vi "Manipulator Panel - UNTOUCHED.vi"() -> ()   [LabVIEW 2012]
uses:
  <vilib>/Platform/TimedLoop/XDataNode/timing_clust.ctl
  <vilib>/Platform/TimedLoop/XDataNode/nitl_modes.ctl
  <vilib>/Platform/TimedLoop/XDataNode/wakeup.ctl
  <vilib>/Platform/TimedLoop/XDataNode/XDataNode.xnode
  <vilib>/Platform/TimedLoop/XDataNode/XDNodeRunTimeDep.lvlib
panel:
  out "Active":bool
  out "Reset":bool
  in  "TCPConRef":refnum<k5>
  out "Turning off in":dbl=10.0
  in  "Power switch\nmanipulator":bool
  in  "Arm Rotate ccw":bool
  in  "Arm Rotate cw":bool
  in  "Claw close":bool
  in  "Claw open":bool
  in  "Arm right":bool
  in  "Arm left":bool
  in  "Lower arm down":bool
  in  "Lower arm up":bool
  in  "Upper arm down":bool
  in  "Upper arm up":bool
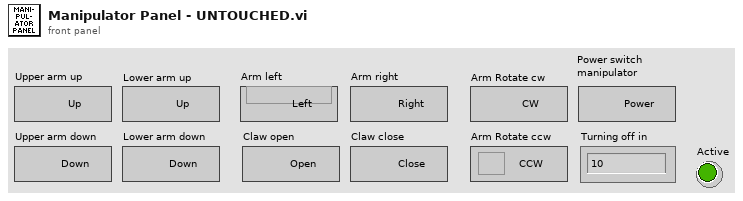
[diagram p1: front panel]
types:
  T1 = typedef "XDNodeRunTimeDep.lvlib/timing_clust.ctl" = cluster{"Expected End [f-1]":u64, "Actual End [f-1]":u64, "Finished Late? [f-1]":bool, "Expected End [i-1]":u64, "Actual End [i-1]":u64, "Finished Late? [i-1]":bool, "Expected Start [i]":u64, "Actual Start [i]":u64, "Expected Start [f]":u64, "Actual Start [f]":u64, "Source Name":string, "Structure Name":string, "Period":i64, "Deadline":i64, "Offset":i64, "Start":i64, "Priority":i32, "Timeout":i32, "Mode":T2, "Wakeup Reason":T3, "Error":errorcluster, "Source Type":string, "Secondary Source Type":string, "Global End Time":u64, "Global Start Time":u64, "Frame Duration":u64, "Iteration Duration":u64, "Assigned CPU":i32, "I/O Scan Engine Mode":u32}
  T2 = typedef "XDNodeRunTimeDep.lvlib/nitl_modes.ctl" = enum32{"No Change", "Process missed periods, maintain original phase", "Discard missed periods, maintain original phase", "Process missed periods, ignore original phase", "Discard missed periods, ignore original phase"}
  T3 = typedef "XDNodeRunTimeDep.lvlib/wakeup.ctl" = enum32{"Normal", "Aborted", "Asynchronous wakeup", "Timing source error", "Timed loop error", "Timeout"}
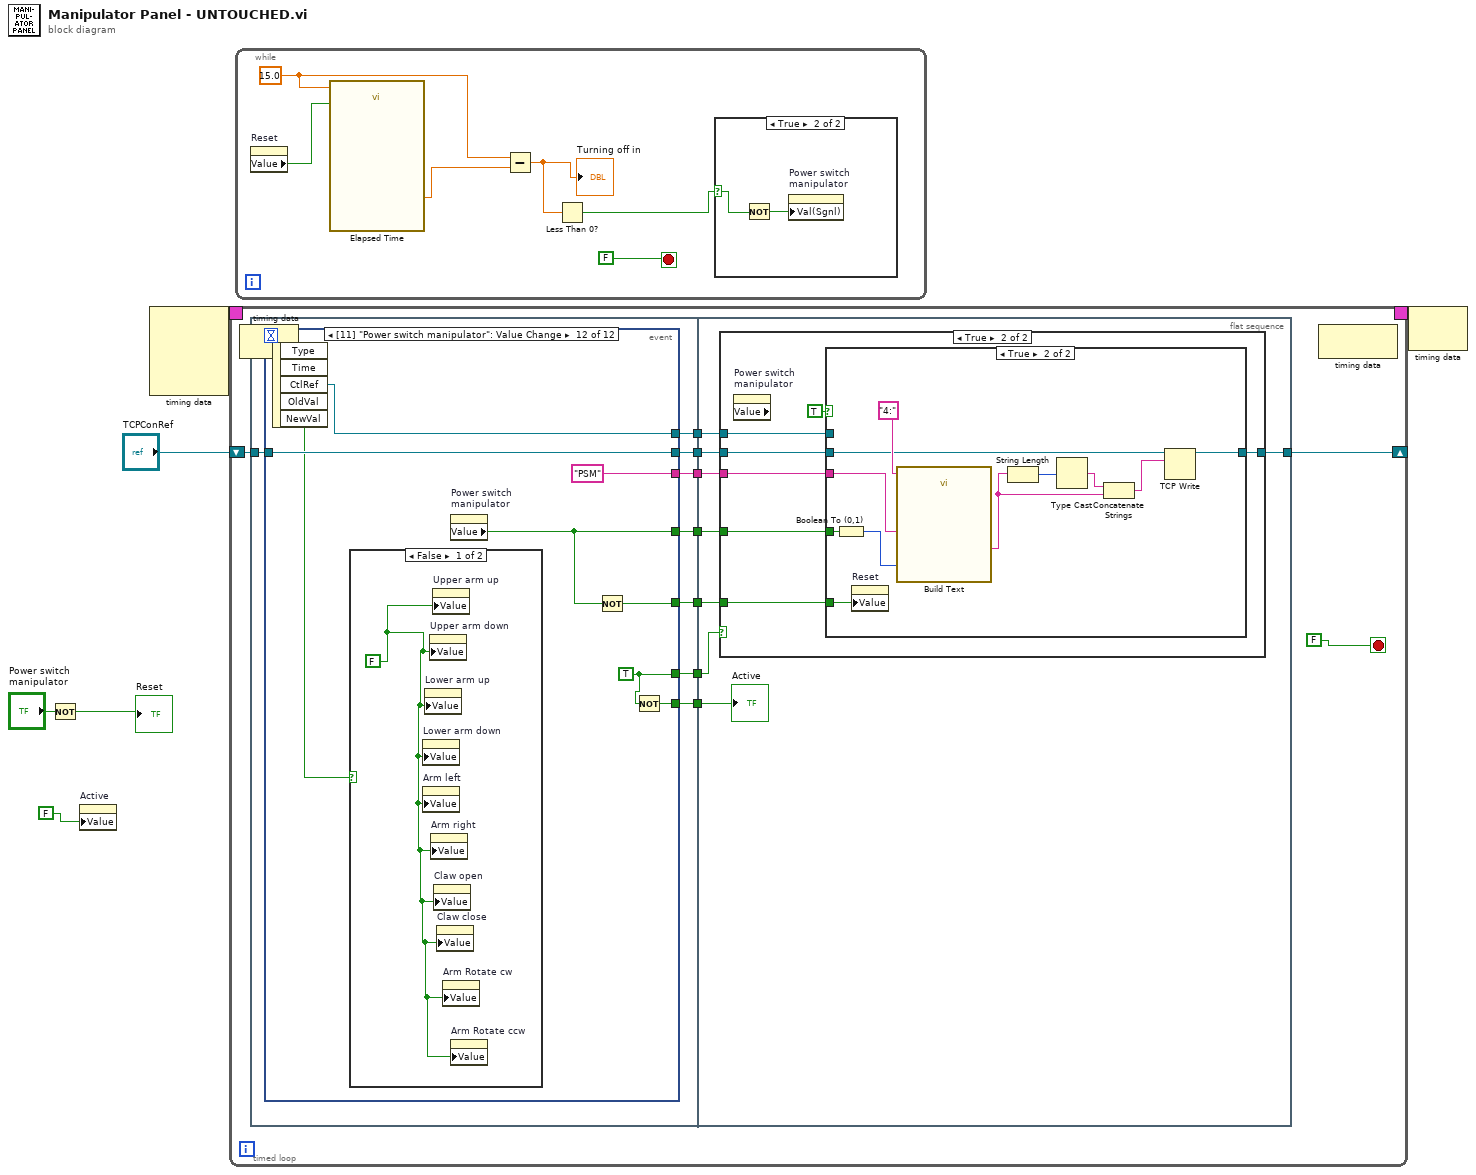
[diagram p0: block diagram]
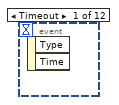
[diagram p2: hidden frame]
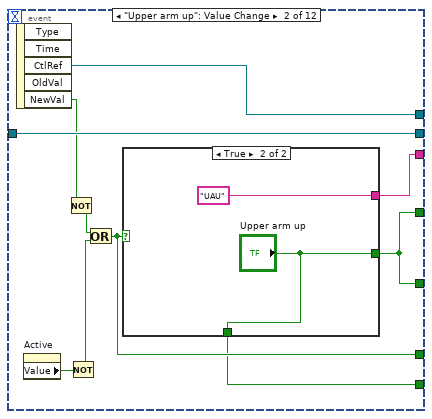
[diagram p3: hidden frame]
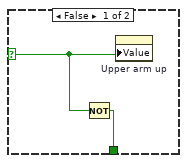
[diagram p4: hidden frame]
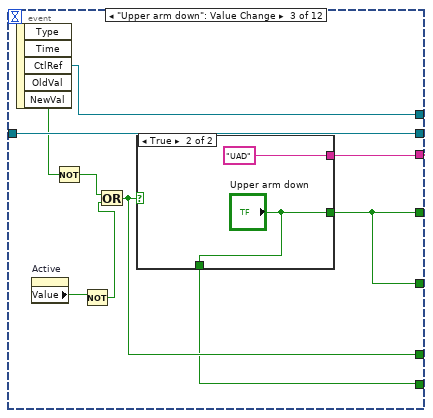
[diagram p5: hidden frame]
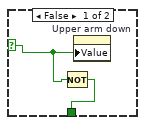
[diagram p6: hidden frame]
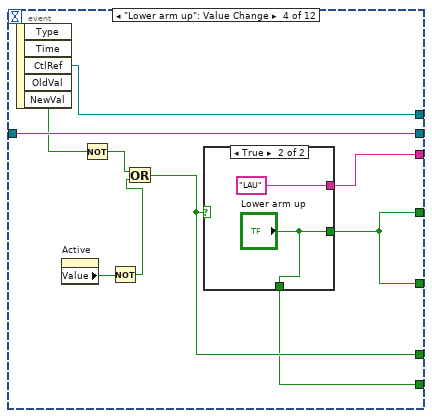
[diagram p7: hidden frame]
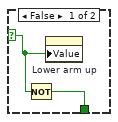
[diagram p8: hidden frame]
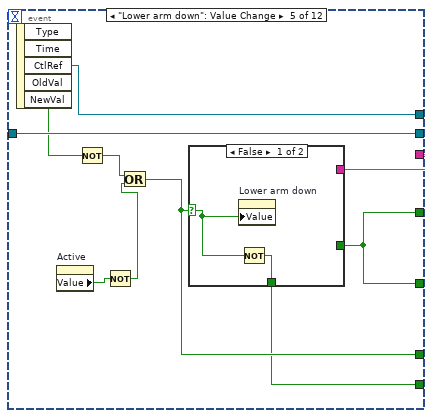
[diagram p9: hidden frame]
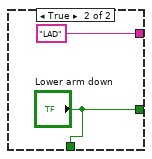
[diagram p10: hidden frame]
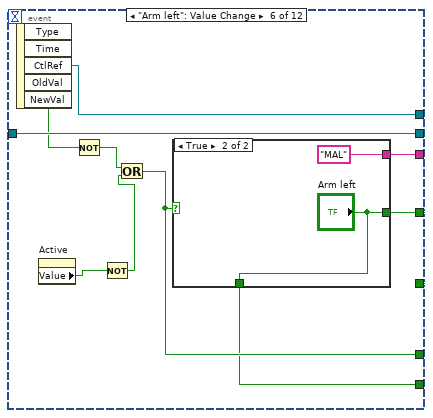
[diagram p11: hidden frame]
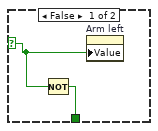
[diagram p12: hidden frame]
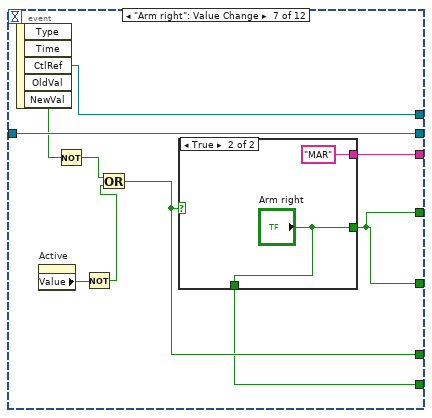
[diagram p13: hidden frame]
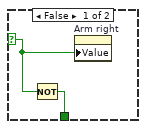
[diagram p14: hidden frame]
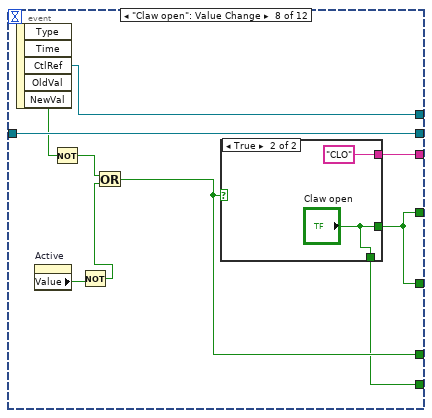
[diagram p15: hidden frame]
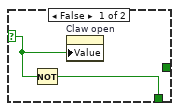
[diagram p16: hidden frame]
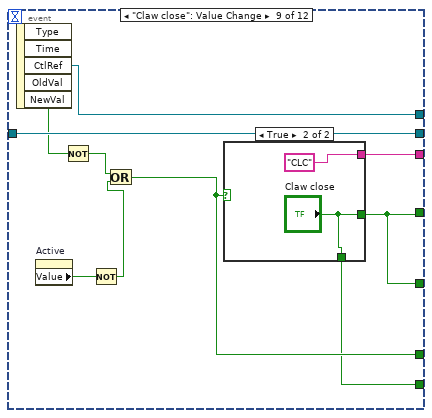
[diagram p17: hidden frame]
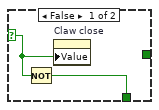
[diagram p18: hidden frame]
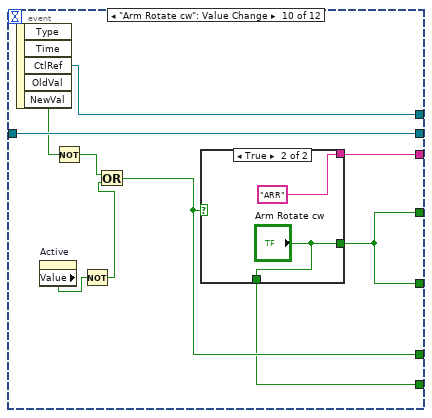
[diagram p19: hidden frame]
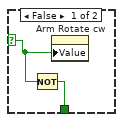
[diagram p20: hidden frame]
diagram:
  n1 = Not(x="Power switch\nmanipulator") -> (.not. x?=→"Reset":bool)
  n2 = property on="Active" class="Bool (strict)"("Value"=FALSE) -> ()  [unwired: 2 in, 2 out]
  n3 = node-c288() -> (w2:T1)  [unwired: 4 in]
  n4 = timed-loop {
    shift-right: [w9] -> _
    shift-left: "TCPConRef" -> [w15]
    timing: w2 -> [_]
    timing-out: [_] -> w1
    stop <- FALSE stop-if-true
    n5 = node-c288() -> ()  [unwired: 1 in, 1 out]
    n6 = flat-sequence {
      tunnel: w15 -> [w26]
      tunnel: [w25] -> w14
      tunnel: [w24] -> w13
      tunnel: [w23] -> w12
      tunnel: [w22] -> w11
      tunnel: [w21] -> w10
      tunnel: [w20] -> w8
      tunnel: [w19] -> w7
      tunnel: w14 -> [w182]
      tunnel: w13 -> [w181]
      tunnel: w12 -> [w180]
      tunnel: w11 -> [w183]
      tunnel: w10 -> [w179]
      tunnel: [w178] -> w9
      tunnel: w8 -> [w177]
      tunnel: w7 -> [w176]
      frame #0 {
        n7 = event shown="[11] \"Power switch manipulator\": Value Change" {
          selector: _ -> [_ _ _ _ _ _ _ _ _ _ _ _]
          dyn-events: _ -> [_ _ _ _ _ _ _ _ _ _ _ _]
          timeout: _ -> [_ _ _ _ _ _ _ _ _ _ _ _]
          tunnel: w26 -> [_ w36 w49 w63 w76 w92 w104 w119 w133 w146 w160 w173]
          tunnel: [_ w36 w49 w63 w76 w92 w104 w119 w133 w146 w160 w173] -> w25
          tunnel: [_ w30 w50 w62 w78 w91 w105 w120 w134 w147 w161 "PSM"] -> w24
          tunnel: [_ w29 w47 w64 w77 w90 w106 w117 w131 w148 w162 w171] -> w23
          tunnel: [_ w29 w47 w64 w77 w90 w106 w117 w131 w148 w162 w172] -> w21
          tunnel: [_ w35 w48 w61 w75 w89 w103 w118 w132 w145 w159 w170] -> w22
          tunnel: [_ w28 w42 w56 w70 w84 w98 w112 w126 w140 w154 w167] -> w20
          tunnel: [_ w27 w41 w55 w69 w83 w97 w111 w125 w139 w153 w168] -> w19
          event Timeout {
            n8 = event-data() -> ()  [unwired: 1 in, 2 out]
          }
          event "Upper arm up": Value Change {
            n9 = event-data() -> ("CtlRef"=w35:refnum<vi>, "NewVal"=w34:bool)  [unwired: 1 in, 3 out]
            n10 = property on="Active" class="Bool (strict)"() -> ("Value"=w33:bool)  [unwired: 2 in, 2 out]
            n11 = Not(x=w34) -> (.not. x?=w31:bool)
            n12 = Not(x=w33) -> (.not. x?=w32:bool)
            n13 = Or(x=w31, y=w32) -> (x .or. y?=w28:bool)
            n14 = case shown="True" w28 {
              selector: w28 -> [w38 _]
              tunnel: [_ "UAU"] -> w30
              tunnel: [_ "Upper arm up"] -> w29
              tunnel: [w37 "Upper arm up"] -> w27
              frame False {
                n15 = Not(x=w38) -> (.not. x?=w37:bool)
                n16 = property on="Upper arm up" class="Bool (strict)"("Value"=w38) -> ()  [unwired: 2 in, 2 out]
              }
              frame True {
              }
            }
          }
          event "Upper arm down": Value Change {
            n17 = event-data() -> ("CtlRef"=w48:refnum<vi>, "NewVal"=w43:bool)  [unwired: 1 in, 3 out]
            n18 = property on="Active" class="Bool (strict)"() -> ("Value"=w46:bool)  [unwired: 2 in, 2 out]
            n19 = Not(x=w43) -> (.not. x?=w44:bool)
            n20 = Not(x=w46) -> (.not. x?=w45:bool)
            n21 = Or(x=w44, y=w45) -> (x .or. y?=w42:bool)
            n22 = case shown="True" w42 {
              selector: w42 -> [w52 _]
              tunnel: [_ "UAD"] -> w50
              tunnel: [_ "Upper arm down"] -> w47
              tunnel: [w51 "Upper arm down"] -> w41
              frame False {
                n23 = Not(x=w52) -> (.not. x?=w51:bool)
                n24 = property on="Upper arm down" class="Bool (strict)"("Value"=w52) -> ()  [unwired: 2 in, 2 out]
              }
              frame True {
              }
            }
          }
          event "Lower arm up": Value Change {
            n25 = event-data() -> ("CtlRef"=w61:refnum<vi>, "NewVal"=w60:bool)  [unwired: 1 in, 3 out]
            n26 = property on="Active" class="Bool (strict)"() -> ("Value"=w57:bool)  [unwired: 2 in, 2 out]
            n27 = Not(x=w60) -> (.not. x?=w59:bool)
            n28 = Not(x=w57) -> (.not. x?=w58:bool)
            n29 = Or(x=w59, y=w58) -> (x .or. y?=w56:bool)
            n30 = case shown="True" w56 {
              selector: w56 -> [w66 _]
              tunnel: [_ "Lower arm up"] -> w64
              tunnel: [_ "LAU"] -> w62
              tunnel: [w65 "Lower arm up"] -> w55
              frame False {
                n31 = Not(x=w66) -> (.not. x?=w65:bool)
                n32 = property on="Lower arm up" class="Bool (strict)"("Value"=w66) -> ()  [unwired: 2 in, 2 out]
              }
              frame True {
              }
            }
          }
          event "Lower arm down": Value Change {
            n33 = event-data() -> ("CtlRef"=w75:refnum<vi>, "NewVal"=w71:bool)  [unwired: 1 in, 3 out]
            n34 = property on="Active" class="Bool (strict)"() -> ("Value"=w74:bool)  [unwired: 2 in, 2 out]
            n35 = Not(x=w71) -> (.not. x?=w72:bool)
            n36 = Not(x=w74) -> (.not. x?=w73:bool)
            n37 = Or(x=w72, y=w73) -> (x .or. y?=w70:bool)
            n38 = case shown="False" w70 {
              selector: w70 -> [w79 _]
              tunnel: [_ "LAD"] -> w78
              tunnel: [_ "Lower arm down"] -> w77
              tunnel: [w80 "Lower arm down"] -> w69
              frame False {
                n39 = property on="Lower arm down" class="Bool (strict)"("Value"=w79) -> ()  [unwired: 2 in, 2 out]
                n40 = Not(x=w79) -> (.not. x?=w80:bool)
              }
              frame True {
              }
            }
          }
          event "Arm left": Value Change {
            n41 = event-data() -> ("CtlRef"=w89:refnum<vi>, "NewVal"=w87:bool)  [unwired: 1 in, 3 out]
            n42 = property on="Active" class="Bool (strict)"() -> ("Value"=w88:bool)  [unwired: 2 in, 2 out]
            n43 = Not(x=w87) -> (.not. x?=w86:bool)
            n44 = Not(x=w88) -> (.not. x?=w85:bool)
            n45 = Or(x=w86, y=w85) -> (x .or. y?=w84:bool)
            n46 = case shown="True" w84 {
              selector: w84 -> [w94 _]
              tunnel: [_ "MAL"] -> w91
              tunnel: [_ "Arm left"] -> w90
              tunnel: [w93 "Arm left"] -> w83
              frame False {
                n47 = Not(x=w94) -> (.not. x?=w93:bool)
                n48 = property on="Arm left" class="Bool (strict)"("Value"=w94) -> ()  [unwired: 2 in, 2 out]
              }
              frame True {
              }
            }
          }
          event "Arm right": Value Change {
            n49 = event-data() -> ("CtlRef"=w103:refnum<vi>, "NewVal"=w100:bool)  [unwired: 1 in, 3 out]
            n50 = property on="Active" class="Bool (strict)"() -> ("Value"=w99:bool)  [unwired: 2 in, 2 out]
            n51 = Not(x=w100) -> (.not. x?=w101:bool)
            n52 = Not(x=w99) -> (.not. x?=w102:bool)
            n53 = Or(x=w101, y=w102) -> (x .or. y?=w98:bool)
            n54 = case shown="True" w98 {
              selector: w98 -> [w108 _]
              tunnel: [_ "Arm right"] -> w106
              tunnel: [_ "MAR"] -> w105
              tunnel: [w107 "Arm right"] -> w97
              frame False {
                n55 = Not(x=w108) -> (.not. x?=w107:bool)
                n56 = property on="Arm right" class="Bool (strict)"("Value"=w108) -> ()  [unwired: 2 in, 2 out]
              }
              frame True {
              }
            }
          }
          event "Claw open": Value Change {
            n57 = event-data() -> ("CtlRef"=w118:refnum<vi>, "NewVal"=w116:bool)  [unwired: 1 in, 3 out]
            n58 = property on="Active" class="Bool (strict)"() -> ("Value"=w113:bool)  [unwired: 2 in, 2 out]
            n59 = Not(x=w116) -> (.not. x?=w115:bool)
            n60 = Not(x=w113) -> (.not. x?=w114:bool)
            n61 = Or(x=w115, y=w114) -> (x .or. y?=w112:bool)
            n62 = case shown="True" w112 {
              selector: w112 -> [w121 _]
              tunnel: [_ "CLO"] -> w120
              tunnel: [_ "Claw open"] -> w117
              tunnel: [w122 "Claw open"] -> w111
              frame False {
                n63 = Not(x=w121) -> (.not. x?=w122:bool)
                n64 = property on="Claw open" class="Bool (strict)"("Value"=w121) -> ()  [unwired: 2 in, 2 out]
              }
              frame True {
              }
            }
          }
          event "Claw close": Value Change {
            n65 = event-data() -> ("CtlRef"=w132:refnum<vi>, "NewVal"=w127:bool)  [unwired: 1 in, 3 out]
            n66 = property on="Active" class="Bool (strict)"() -> ("Value"=w128:bool)  [unwired: 2 in, 2 out]
            n67 = Not(x=w127) -> (.not. x?=w130:bool)
            n68 = Not(x=w128) -> (.not. x?=w129:bool)
            n69 = Or(x=w130, y=w129) -> (x .or. y?=w126:bool)
            n70 = case shown="True" w126 {
              selector: w126 -> [w136 _]
              tunnel: [_ "CLC"] -> w134
              tunnel: [_ "Claw close"] -> w131
              tunnel: [w135 "Claw close"] -> w125
              frame False {
                n71 = Not(x=w136) -> (.not. x?=w135:bool)
                n72 = property on="Claw close" class="Bool (strict)"("Value"=w136) -> ()  [unwired: 2 in, 2 out]
              }
              frame True {
              }
            }
          }
          event "Arm Rotate cw": Value Change {
            n73 = event-data() -> ("CtlRef"=w145:refnum<vi>, "NewVal"=w142:bool)  [unwired: 1 in, 3 out]
            n74 = property on="Active" class="Bool (strict)"() -> ("Value"=w141:bool)  [unwired: 2 in, 2 out]
            n75 = Not(x=w142) -> (.not. x?=w143:bool)
            n76 = Not(x=w141) -> (.not. x?=w144:bool)
            n77 = Or(x=w143, y=w144) -> (x .or. y?=w140:bool)
            n78 = case shown="True" w140 {
              selector: w140 -> [w150 _]
              tunnel: [_ "Arm Rotate cw"] -> w148
              tunnel: [_ "ARR"] -> w147
              tunnel: [w149 "Arm Rotate cw"] -> w139
              frame False {
                n79 = Not(x=w150) -> (.not. x?=w149:bool)
                n80 = property on="Arm Rotate cw" class="Bool (strict)"("Value"=w150) -> ()  [unwired: 2 in, 2 out]
              }
              frame True {
              }
            }
          }
          event "Arm Rotate ccw": Value Change {
            n81 = event-data() -> ("CtlRef"=w159:refnum<vi>, "NewVal"=w156:bool)  [unwired: 1 in, 3 out]
            n82 = property on="Active" class="Bool (strict)"() -> ("Value"=w155:bool)  [unwired: 2 in, 2 out]
            n83 = Not(x=w156) -> (.not. x?=w157:bool)
            n84 = Not(x=w155) -> (.not. x?=w158:bool)
            n85 = Or(x=w157, y=w158) -> (x .or. y?=w154:bool)
            n86 = case shown="True" w154 {
              selector: w154 -> [w164 _]
              tunnel: [_ "Arm Rotate ccw"] -> w162
              tunnel: [_ "ARL"] -> w161
              tunnel: [w163 "Arm Rotate ccw"] -> w153
              frame False {
                n87 = Not(x=w164) -> (.not. x?=w163:bool)
                n88 = property on="Arm Rotate ccw" class="Bool (strict)"("Value"=w164) -> ()  [unwired: 2 in, 2 out]
              }
              frame True {
              }
            }
          }
          event "Power switch\nmanipulator": Value Change {
            w167 = TRUE
            n89 = event-data() -> ("CtlRef"=w170:refnum<vi>, "NewVal"=w169:bool)  [unwired: 1 in, 3 out]
            n90 = case shown="False" w169 {
              frame False {
                w175 = FALSE
                n91 = property on="Lower arm down" class="Bool (strict)"("Value"=w175) -> ()  [unwired: 2 in, 2 out]
                n92 = property on="Arm left" class="Bool (strict)"("Value"=w175) -> ()  [unwired: 2 in, 2 out]
                n93 = property on="Lower arm up" class="Bool (strict)"("Value"=w175) -> ()  [unwired: 2 in, 2 out]
                n94 = property on="Upper arm down" class="Bool (strict)"("Value"=w175) -> ()  [unwired: 2 in, 2 out]
                n95 = property on="Arm right" class="Bool (strict)"("Value"=w175) -> ()  [unwired: 2 in, 2 out]
                n96 = property on="Upper arm up" class="Bool (strict)"("Value"=w175) -> ()  [unwired: 2 in, 2 out]
                n97 = property on="Claw open" class="Bool (strict)"("Value"=w175) -> ()  [unwired: 2 in, 2 out]
                n98 = property on="Claw close" class="Bool (strict)"("Value"=w175) -> ()  [unwired: 2 in, 2 out]
                n99 = property on="Arm Rotate cw" class="Bool (strict)"("Value"=w175) -> ()  [unwired: 2 in, 2 out]
                n100 = property on="Arm Rotate ccw" class="Bool (strict)"("Value"=w175) -> ()  [unwired: 2 in, 2 out]
              }
              frame True {
              }
            }
            n101 = property on="Power switch\nmanipulator" class="Bool (strict)"() -> ("Value"=w171:bool)  [unwired: 2 in, 2 out]
            n102 = Not(x=w171) -> (.not. x?=w172:bool)
            n103 = Not(x=w167) -> (.not. x?=w168:bool)
          }
        }
      }
      frame #1 {
        n104 = case shown="True" w177 {
          tunnel: w183 -> [_ w191]
          tunnel: w182 -> [w184 w190]
          tunnel: w181 -> [_ w189]
          tunnel: w180 -> [_ w188]
          tunnel: w179 -> [_ w187]
          tunnel: [w184 w186] -> w178
          frame False {
          }
          frame True {
            n105 = property on="Power switch\nmanipulator" class="Bool (strict)" props=["Value"]() -> ()  [unwired: 2 in, 3 out]
            n106 = case shown="True" TRUE {
              tunnel: w190 -> [w193 w204]
              tunnel: [w193 w203] -> w186
              tunnel: w189 -> [_ w212]
              tunnel: w188 -> [_ w207]
              tunnel: w191 -> [w194 _]
              tunnel: w187 -> [_ w205]
              frame False {
                n107 = control-ref of="Power switch\nmanipulator"() -> (w195:refnum<vi>)
                n108 = Not Equal?(x=w194, y=w195) -> (x != y?=w192:bool)
                n109 = case shown="True" w192 {
                  tunnel: w194 -> [w198 w200]
                  frame False {
                    n110 = property class="Bool (strict)"(reference=w198) -> ("Value"=w197:bool)  [unwired: 1 in, 2 out]
                    n111 = Not(x=w197) -> (.not. x?=w196:bool)
                    n112 = property on="Reset" class="Bool (strict)"("Value"=w196) -> ()  [unwired: 2 in, 2 out]
                  }
                  frame True {
                    n113 = property class="Bool (strict)"(reference=w200, "Value"=FALSE) -> ()  [unwired: 1 in, 2 out]
                    n114 = One Button Dialog(message="You must start the\nmanipulator engine first") -> ()  [unwired: 1 in, 1 out]
                  }
                }
              }
              frame True {
                n115 = Boolean To (0,1)(Boolean=w207) -> (0, 1=w206:i16)
                n116 = property on="Reset" class="Bool (strict)"("Value"=w205) -> ()  [unwired: 2 in, 2 out]
                n117 = call "Build Text"("Beginning Text"="4:", "ControlID"=w212, "Bool"=w206) -> ("Result"=w208:string)  [unwired: 11 in, 1 out]
                n118 = String Length(string=w208) -> (length=w210:i32)
                n119 = Type Cast(x=w210) -> (*(type *) &x=w209:string)  [unwired: 1 in]
                n120 = Concatenate Strings(w209, w208) -> (w202:string)
                n121 = TCP Write(connection ID=w204, data in=w202) -> (connection ID out=w203:refnum<k5>)  [unwired: 2 in, 2 out]
              }
            }
          }
        }
        "Active" <- w176
      }
    }
    n122 = node-c288() -> ()  [unwired: 1 in, 1 out]
  }
  n123 = while {
    stop <- FALSE stop-if-true
    w218 = 15.0
    n124 = property on="Reset" class="Bool (strict)"() -> ("Value"=w215:bool)  [unwired: 2 in, 2 out]
    n125 = call "Elapsed Time"("Time Target (s)"=w218, "Reset"=w215) -> ("Elapsed Time (s)"=w217:dbl)  [unwired: 10 in, 7 out]
    n126 = Subtract(x=w218, y=w217) -> (x-y=w214:dbl)
    "Turning off in" <- w214
    n127 = Less Than 0?(x=w214) -> (x < 0?=w213:bool)
    n128 = case shown="True" w213 {
      selector: w213 -> [_ w219]
      frame False {
      }
      frame True {
        n129 = Not(x=w219) -> (.not. x?=w220:bool)
        n130 = property on="Power switch\nmanipulator" class="Bool (strict)"("Val(Sgnl)"=w220) -> ()  [unwired: 2 in, 2 out]
      }
    }
  }
  n131 = node-c288(w1) -> ()  [unwired: 1 out]
